vi "Main_18b.vi"() -> ()   [LabVIEW 2023]
uses:
  Cluster_Location.ctl
panel:
  out "MAX Surfaces":i32
  out "number of Blocks":i32
  in  "Example 2":string="2,2,2\n1,2,2\n3,2,2\n2,1,2\n2,3,2\n2,2,1\n2,2,3\n2,2,4\n2,2,6\n1,2,5\n3,2,5\n2,1,5\n2,3,5"
  out "z":i32
  out "x":i32
  out "y":i32
  out "Answer":i32
  in  "Puzzle":string="8,17,5\n6,17,7\n8,9,2\n13,5,16\n5,3,9\n19,4,10\n5,14,5\n3,5,12\n4,6,13\n11,9,3\n11,2,14\n3,14,10\n12,1,11\n16,16,13\n1,9,10\n11,9,19\n15,15,12\n10,4,6\n4,12,17\n17,6,15\n19,14,13\n9,13,2\n18,8,14\n17,7,15\n10,5,17\n14,8,17\n11,19,13\n13,3,14\n8,5,10\n8,16,6\n10,7,20\n7,17,5\n12,18,13\n4,8,13\n3,13,13\n4,3,11\n4,9,15\n17,6,7\n13,5,14\n3,12,7\n13,18,7\n1,9,11\n17,8,15\n12,8,2\n4,9,6\n3,7,12\n8,13,4\n3,8,7\n14,7,3\n16,7,14\n17,5,12\n13,8,2\n17,5,5\n16,5,13\n5,4,13\n6,1,9\n1,11,10\n5,13,5\n10,17,5\n6,3,9\n15,6,7\n11,15,17\n18,6,12\n8,3,11\n14,7,14\n10,6,18\n12,11,4\n3,7,15\n7,3,10\n18,8,13\n16,11,19\n11,3,11\n3,15,14\n16,14,3\n19,10,8\n8,13,18\n15,10,3\n20,7,12\n13,15,16\n18,10,9\n10,2,7\n16,5,12\n6,10,18\n12,19,13\n6,5,6\n14,2,8\n4,16,9\n6,17,9\n15,6,5\n9,4,3\n11,7,2\n19,9,6\n14,12,2\n15,6,18\n18,13,7\n5,6,6\n20,11,14\n19,10,10\n18,10,6\n6,10,5\n16,10,18\n3,9,7\n13,2,7\n14,9,19\n9,14,19\n7,18,6\n8,9,19\n11,1,13\n15,17,10\n2,12,13\n5,17,14\n18,9,11\n15,18,15\n7,3,11\n10,18,6\n17,15,14\n17,7,8\n7,3,14\n7,11,19\n7,9,3\n17,11,6\n16,3,10\n9,18,16\n13,1,10\n15,12,16\n14,12,20\n11,2,8\n18,5,9\n11,16,3\n18,10,7\n4,12,6\n5,11,18\n3,14,14\n16,4,12\n8,3,4\n6,14,3\n17,9,18\n2,11,7\n19,15,12\n13,17,15\n10,7,3\n1,11,8\n18,12,16\n18,12,9\n7,4,4\n12,2,7\n7,14,15\n15,13,3\n3,7,11\n12,17,10\n17,5,14\n5,18,11\n5,4,11\n4,15,15\n8,19,12\n18,12,10\n9,3,11\n3,14,12\n18,7,16\n10,9,19\n16,3,11\n15,11,17\n18,7,12\n9,8,19\n3,15,12\n17,4,12\n5,16,7\n8,4,5\n2,7,11\n5,15,17\n9,20,12\n5,11,4\n4,5,9\n4,15,11\n14,14,5\n11,3,6\n12,3,15\n5,6,10\n5,9,5\n18,15,12\n4,12,5\n19,9,15\n4,6,11\n1,14,9\n5,16,15\n9,3,7\n16,10,4\n17,12,7\n18,8,7\n14,5,9\n6,6,14\n5,14,15\n6,7,3\n18,15,15\n12,7,17\n5,14,16\n6,11,3\n6,10,16\n3,7,8\n10,7,4\n8,8,3\n11,4,5\n16,13,18\n13,6,4\n10,17,16\n3,16,10\n10,19,13\n15,5,16\n9,19,6\n9,13,4\n17,16,7\n12,4,15\n7,4,15\n18,17,10\n14,17,7\n13,15,19\n4,10,15\n13,18,17\n14,19,10\n18,10,15\n14,18,8\n16,4,13\n17,14,9\n14,17,5\n6,7,4\n5,9,16\n5,14,17\n14,19,11\n6,18,7\n14,9,18\n17,7,16\n4,10,16\n11,13,3\n3,10,16\n8,9,18\n13,3,15\n17,8,6\n3,13,9\n5,17,10\n14,15,3\n15,5,15\n16,17,15\n9,20,8\n8,2,13\n20,8,8\n17,14,12\n5,7,18\n5,10,16\n3,8,11\n3,11,16\n15,7,5\n17,12,18\n10,19,11\n11,2,10\n18,11,6\n5,11,17\n15,10,15\n18,15,9\n7,5,15\n17,8,5\n5,5,6\n17,14,16\n15,11,5\n8,10,19\n3,13,14\n7,3,9\n13,2,8\n17,9,6\n17,16,11\n11,10,18\n12,17,18\n5,3,14\n12,9,2\n5,14,6\n14,15,15\n15,4,9\n8,12,17\n10,9,3\n4,17,9\n1,11,12\n3,14,11\n11,19,9\n12,17,8\n5,5,9\n19,9,12\n16,4,14\n18,10,14\n8,19,13\n11,3,8\n6,6,4\n13,6,18\n6,14,4\n18,6,8\n4,13,15\n11,7,1\n11,7,18\n10,3,7\n14,15,7\n6,16,9\n14,7,19\n12,6,17\n16,12,5\n3,10,7\n7,12,5\n16,10,15\n17,8,11\n10,18,14\n3,11,4\n7,10,19\n10,4,3\n12,16,6\n9,8,1\n10,4,15\n14,4,5\n5,8,16\n8,13,3\n19,10,9\n17,17,13\n4,5,11\n14,5,16\n16,11,17\n17,7,6\n1,10,11\n11,8,16\n4,15,6\n10,19,14\n6,4,9\n18,11,8\n10,4,5\n11,13,19\n13,6,16\n5,10,17\n3,11,5\n18,17,9\n18,14,11\n10,1,7\n15,9,3\n8,6,3\n6,3,12\n12,2,8\n14,16,17\n16,8,4\n15,7,4\n19,15,9\n17,16,9\n7,14,19\n3,10,8\n9,20,13\n8,8,1\n5,12,4\n8,17,15\n17,3,10\n16,8,6\n18,10,5\n15,8,5\n6,12,4\n1,16,10\n15,17,6\n20,11,11\n4,4,14\n9,9,3\n6,15,17\n16,9,17\n12,12,19\n19,8,10\n4,14,17\n9,15,17\n10,3,14\n4,6,7\n2,8,12\n13,2,11\n7,11,2\n10,19,7\n15,10,2\n6,13,3\n11,10,20\n6,12,18\n15,18,13\n10,8,2\n13,5,5\n11,2,9\n6,17,14\n6,8,5\n14,14,16\n6,8,16\n3,12,16\n8,17,18\n12,2,11\n3,15,11\n10,11,2\n11,17,12\n9,15,3\n6,16,17\n18,6,6\n16,12,16\n7,18,12\n17,15,4\n9,12,18\n17,6,6\n11,8,19\n12,8,3\n20,9,14\n4,12,16\n20,11,10\n4,15,8\n4,7,9\n16,7,5\n10,9,18\n2,11,12\n4,13,16\n9,2,10\n16,7,18\n17,11,16\n6,15,4\n7,18,7\n6,9,19\n8,15,4\n5,16,14\n2,10,7\n8,12,4\n14,18,13\n12,14,17\n15,11,19\n6,13,16\n14,7,18\n19,11,7\n6,17,16\n10,11,3\n7,20,13\n10,18,7\n8,17,6\n4,7,16\n8,3,15\n2,10,9\n5,3,13\n17,10,15\n9,4,6\n8,19,11\n9,16,4\n14,8,19\n13,12,15\n4,13,17\n14,16,5\n5,6,16\n14,13,17\n18,7,13\n12,3,6\n6,4,14\n10,4,9\n3,10,6\n8,19,9\n11,7,19\n19,12,14\n18,9,10\n16,10,17\n16,6,16\n17,15,15\n7,18,11\n1,10,12\n12,4,13\n8,5,5\n20,10,12\n9,18,8\n18,13,9\n8,17,4\n18,7,6\n7,13,4\n15,17,14\n11,17,17\n4,11,16\n7,5,17\n8,15,17\n14,18,6\n15,12,3\n2,7,13\n11,5,5\n19,14,11\n15,18,9\n11,18,5\n7,6,6\n10,11,19\n8,14,3\n6,13,17\n12,5,15\n16,9,3\n3,5,6\n10,4,16\n14,13,19\n3,6,12\n9,15,14\n17,13,7\n7,19,11\n8,14,16\n3,17,12\n9,11,18\n18,14,7\n17,17,9\n8,13,2\n4,16,15\n11,15,4\n8,4,9\n13,6,17\n4,7,12\n13,3,10\n6,5,9\n5,6,5\n15,14,5\n11,4,6\n4,17,13\n3,11,11\n16,13,5\n12,9,1\n13,9,18\n8,17,9\n5,11,15\n16,14,5\n13,11,19\n10,16,17\n9,12,3\n3,12,10\n6,9,4\n5,13,15\n11,6,18\n16,4,9\n7,12,3\n18,12,6\n10,16,18\n14,6,18\n4,5,7\n6,8,18\n15,10,18\n8,3,13\n10,5,18\n3,6,15\n14,6,16\n14,6,17\n12,10,3\n2,14,12\n18,5,10\n15,9,17\n8,6,18\n3,16,14\n10,13,4\n10,15,19\n4,8,17\n13,6,5\n3,6,10\n12,20,10\n11,6,4\n18,4,11\n17,9,11\n15,4,13\n9,17,5\n6,3,11\n11,19,6\n17,6,14\n7,7,18\n8,10,2\n9,3,15\n4,16,13\n11,5,15\n3,6,13\n8,15,18\n14,3,14\n6,5,14\n5,12,18\n8,3,12\n15,4,16\n6,6,15\n16,16,9\n15,3,14\n8,14,18\n10,17,6\n5,9,6\n15,8,16\n18,6,5\n15,13,4\n15,16,5\n10,7,5\n9,7,18\n16,3,13\n4,8,4\n11,11,19\n17,13,12\n17,11,15\n4,13,14\n10,2,6\n4,10,4\n10,3,6\n9,16,17\n8,1,9\n14,20,9\n3,7,14\n8,18,16\n3,11,14\n16,14,15\n3,10,9\n17,12,12\n3,14,5\n10,16,3\n5,15,13\n15,16,7\n12,16,19\n2,12,11\n2,13,10\n13,18,14\n16,15,18\n2,10,15\n2,8,8\n6,7,6\n13,5,17\n6,4,15\n9,17,6\n5,16,13\n11,5,18\n7,17,10\n17,6,5\n14,4,12\n8,12,20\n2,15,10\n18,6,13\n12,19,16\n19,7,5\n19,9,14\n10,13,18\n6,11,19\n10,14,3\n19,7,11\n7,18,16\n14,9,2\n12,4,5\n15,14,6\n5,9,17\n11,14,2\n15,13,18\n16,16,8\n2,5,9\n2,8,10\n16,5,6\n6,18,10\n12,18,15\n4,14,12\n15,8,17\n18,9,9\n11,10,1\n12,3,3\n9,19,9\n8,5,13\n20,14,12\n16,5,15\n1,12,10\n19,15,11\n13,17,10\n12,2,5\n3,5,10\n7,6,5\n5,7,4\n9,6,18\n16,17,12\n7,8,19\n17,11,12\n10,18,15\n13,16,15\n2,12,14\n8,12,2\n14,18,7\n17,5,9\n3,13,5\n10,14,19\n3,8,13\n16,15,3\n11,6,20\n3,14,8\n14,8,18\n7,17,12\n4,13,5\n17,7,5\n8,7,17\n14,4,6\n17,12,4\n13,3,6\n10,12,3\n9,21,11\n17,11,13\n2,16,13\n7,5,3\n14,16,16\n17,15,6\n14,3,13\n11,3,13\n16,16,15\n13,2,13\n17,14,15\n12,2,15\n17,14,11\n10,14,4\n6,8,4\n16,7,15\n11,4,17\n17,17,11\n12,4,17\n6,9,15\n12,9,20\n16,11,5\n18,5,7\n8,11,18\n15,12,6\n12,13,3\n7,15,3\n5,11,3\n11,16,8\n16,17,14\n4,8,7\n14,5,7\n4,13,18\n15,17,7\n16,15,17\n14,20,11\n10,6,14\n12,19,10\n13,3,16\n13,18,8\n13,19,10\n10,10,3\n9,2,8\n6,16,16\n6,16,7\n13,17,5\n3,8,12\n12,13,17\n13,19,12\n19,13,8\n6,10,17\n16,16,7\n7,14,6\n5,15,6\n13,1,12\n7,3,13\n11,17,6\n13,15,3\n10,2,12\n14,2,13\n19,11,6\n8,8,17\n4,6,6\n4,16,10\n4,5,12\n14,19,14\n17,15,16\n11,15,18\n10,15,3\n8,2,10\n15,9,8\n17,13,16\n2,13,14\n15,7,6\n10,12,20\n4,17,14\n12,6,16\n18,7,7\n5,9,4\n16,15,7\n18,16,10\n10,2,10\n13,17,17\n15,6,12\n10,7,2\n11,0,12\n13,2,6\n17,9,5\n10,16,5\n19,10,13\n7,11,16\n5,17,13\n8,18,13\n15,7,19\n3,12,8\n7,18,15\n12,17,3\n16,5,16\n9,16,16\n14,5,15\n8,2,9\n7,16,7\n12,5,16\n19,8,15\n17,10,16\n9,5,6\n12,7,4\n3,4,9\n11,14,19\n12,12,1\n15,12,4\n16,12,17\n18,10,12\n19,12,6\n15,8,15\n12,19,14\n3,8,6\n14,2,12\n11,5,4\n10,5,3\n9,11,3\n7,12,19\n3,5,7\n20,7,11\n15,3,12\n13,4,9\n13,14,2\n17,13,14\n16,4,11\n10,3,17\n15,16,8\n18,16,8\n4,14,14\n11,19,8\n5,11,6\n9,3,16\n10,17,7\n13,9,19\n5,13,8\n12,4,4\n8,13,1\n7,2,11\n6,6,5\n9,5,3\n12,14,3\n14,3,11\n10,6,4\n8,16,18\n10,18,17\n9,7,2\n6,5,8\n10,2,13\n17,8,16\n6,3,10\n7,13,18\n8,18,14\n4,9,17\n12,7,19\n3,12,11\n16,16,14\n4,14,13\n9,5,5\n4,6,16\n7,16,16\n12,15,17\n19,16,11\n8,9,16\n1,13,13\n16,15,5\n2,11,8\n6,2,12\n9,5,15\n12,2,13\n8,13,19\n15,5,7\n7,19,9\n7,1,8\n17,8,4\n5,5,4\n5,4,12\n11,12,3\n8,15,3\n16,16,12\n16,13,17\n5,6,8\n10,10,2\n4,16,14\n10,8,20\n3,9,16\n5,12,5\n7,16,6\n18,6,14\n6,5,17\n2,7,8\n16,17,11\n12,3,12\n11,4,16\n17,11,5\n13,4,11\n15,6,8\n6,10,6\n11,1,10\n10,19,12\n3,14,13\n12,18,9\n7,15,5\n10,3,9\n10,8,18\n16,14,4\n20,9,9\n10,15,2\n10,5,16\n10,17,4\n14,11,2\n15,9,4\n15,3,9\n15,6,17\n2,9,11\n7,13,17\n6,17,15\n16,12,4\n16,5,7\n11,5,17\n5,12,7\n10,3,13\n6,10,4\n17,10,4\n6,4,10\n14,18,14\n12,18,10\n13,18,6\n15,6,13\n15,16,12\n16,6,12\n17,10,7\n17,10,5\n1,9,12\n3,9,5\n17,15,7\n13,13,4\n4,5,13\n15,12,2\n13,4,4\n15,13,17\n19,12,10\n15,18,7\n12,17,17\n16,7,4\n19,7,12\n3,12,5\n11,19,12\n10,20,9\n13,15,18\n18,6,11\n9,1,10\n12,8,20\n18,13,10\n2,12,15\n3,6,11\n14,8,16\n7,10,5\n4,13,6\n10,14,1\n7,12,18\n10,18,11\n2,11,13\n6,6,6\n17,4,8\n13,4,16\n5,14,9\n18,12,5\n4,12,12\n18,15,11\n12,17,4\n17,7,11\n12,17,15\n13,10,1\n2,15,9\n4,10,5\n6,14,6\n15,7,7\n6,16,12\n15,9,2\n12,2,12\n9,4,5\n3,14,7\n9,15,5\n4,7,8\n8,16,17\n19,6,9\n19,8,7\n13,3,9\n14,13,15\n7,17,14\n8,4,12\n13,18,9\n6,5,15\n17,5,6\n13,13,3\n13,17,13\n13,6,2\n11,3,9\n3,8,14\n7,4,8\n4,14,6\n8,5,18\n13,7,18\n13,7,3\n14,11,17\n7,5,16\n13,3,12\n19,12,15\n14,3,5\n17,11,18\n9,3,10\n15,7,3\n2,9,12\n6,18,9\n3,6,9\n13,19,7\n18,11,7\n3,15,8\n2,12,12\n16,15,11\n4,4,11\n6,7,11\n1,10,13\n15,3,11\n14,18,10\n6,9,18\n18,9,15\n12,19,11\n7,6,7\n3,12,18\n3,11,9\n14,17,6\n16,16,11\n18,14,14\n8,20,11\n18,6,7\n15,6,16\n5,9,3\n14,2,14\n10,7,18\n7,4,17\n20,6,9\n15,5,10\n15,4,12\n20,10,15\n6,12,2\n10,4,4\n5,15,15\n5,16,10\n6,11,2\n10,13,2\n7,15,4\n15,16,4\n16,5,8\n4,6,15\n8,5,14\n4,17,12\n6,14,5\n11,17,7\n15,14,15\n17,12,5\n6,18,13\n16,17,9\n7,7,16\n4,6,9\n7,10,3\n16,14,12\n19,12,12\n15,17,9\n13,2,12\n6,9,3\n12,3,9\n15,14,3\n14,14,19\n14,8,3\n9,8,18\n4,13,7\n10,4,8\n8,1,7\n5,5,13\n14,3,16\n6,20,9\n6,15,18\n5,14,18\n19,9,8\n5,2,12\n16,8,15\n10,3,8\n13,15,4\n8,16,3\n13,13,2\n14,18,12\n16,5,14\n11,14,18\n5,7,5\n8,9,20\n9,8,3\n16,16,6\n13,20,9\n11,18,14\n15,13,5\n11,14,17\n12,17,6\n10,17,15\n6,8,15\n2,7,12\n12,20,13\n9,14,17\n12,16,5\n10,19,6\n7,7,4\n1,11,11\n19,6,10\n15,14,4\n19,13,12\n4,7,6\n9,2,12\n9,19,15\n18,14,16\n11,10,2\n13,16,4\n17,12,15\n2,10,10\n2,13,13\n5,10,3\n10,16,7\n11,19,10\n17,14,8\n12,12,20\n7,5,8\n11,8,20\n5,15,8\n3,9,8\n13,5,13\n17,15,10\n14,11,19\n15,5,4\n15,3,8\n15,4,6\n4,15,14\n17,11,17\n12,6,15\n3,16,7\n4,11,5\n13,10,3\n7,14,3\n6,17,12\n14,16,4\n4,16,12\n4,14,5\n14,19,9\n19,13,9\n10,10,19\n11,11,1\n18,16,12\n17,17,8\n10,12,2\n7,18,8\n1,8,12\n19,8,6\n4,6,8\n13,14,17\n20,10,8\n19,7,7\n12,3,14\n2,9,8\n5,17,11\n11,8,2\n7,18,9\n8,7,3\n9,15,18\n10,6,16\n7,16,3\n15,8,18\n11,14,3\n17,13,6\n11,8,18\n14,5,5\n17,16,14\n17,13,4\n9,7,17\n13,5,6\n14,3,12\n3,13,16\n11,3,7\n16,10,16\n11,16,4\n7,3,15\n5,16,11\n20,9,10\n18,8,9\n19,8,8\n20,9,13\n11,16,16\n15,11,2\n1,13,12\n14,13,4\n12,18,11\n14,16,3\n11,5,11\n17,7,13\n15,11,18\n7,17,9\n5,5,14\n11,9,2\n4,7,14\n7,17,15\n5,12,17\n3,8,15\n18,10,16\n15,4,11\n12,5,6\n19,11,11\n11,18,17\n18,13,16\n7,4,7\n7,5,6\n13,10,19\n13,18,10\n16,15,16\n5,7,15\n12,12,2\n2,14,8\n20,9,11\n4,7,11\n5,11,12\n16,16,10\n3,17,9\n2,9,9\n17,18,9\n3,12,15\n5,3,11\n15,4,15\n20,10,14\n19,13,11\n5,13,18\n17,9,4\n13,12,17\n3,15,13\n14,10,6\n16,16,5\n5,8,17\n15,3,6\n18,15,10\n15,6,6\n18,11,14\n17,12,13\n4,6,14\n5,14,3\n15,5,6\n11,15,3\n12,2,9\n14,3,15\n17,12,16\n15,17,13\n13,12,1\n14,3,10\n18,9,14\n12,17,11\n16,11,15\n18,8,6\n3,12,6\n3,9,6\n7,16,8\n16,12,15\n18,8,10\n4,5,10\n12,19,7\n14,2,9\n8,7,6\n12,3,11\n4,7,7\n9,18,14\n4,6,5\n11,17,16\n8,19,10\n12,8,19\n3,17,13\n15,12,18\n4,4,13\n10,19,8\n16,8,17\n9,7,16\n19,14,9\n9,8,2\n16,8,13\n7,5,14\n7,6,4\n18,11,10\n6,4,5\n18,7,14\n18,11,13\n9,6,3\n8,16,15\n7,8,3\n12,9,3\n9,19,7\n8,6,16\n10,4,17\n17,4,14\n11,13,18\n6,8,17\n3,7,17\n16,4,8\n2,10,8\n5,18,8\n9,3,6\n18,9,5\n9,15,19\n3,16,9\n7,6,17\n7,16,17\n12,11,19\n12,10,2\n4,7,10\n6,19,13\n19,11,10\n9,10,1\n12,14,4\n4,9,4\n18,16,9\n5,3,8\n9,18,4\n3,13,6\n16,15,14\n13,8,19\n12,16,14\n8,10,15\n11,21,12\n5,15,5\n8,9,15\n18,11,5\n16,17,8\n10,17,17\n11,8,3\n7,19,12\n14,16,8\n17,15,12\n11,11,4\n7,6,19\n3,16,12\n17,5,10\n11,3,16\n8,15,14\n8,15,5\n2,9,13\n5,11,5\n4,4,8\n12,5,17\n7,5,7\n6,19,11\n4,7,4\n17,9,7\n15,7,16\n9,14,3\n14,4,15\n16,7,17\n3,12,9\n17,9,16\n8,18,10\n11,16,5\n10,18,8\n14,5,6\n12,15,16\n10,6,19\n14,7,17\n2,14,11\n8,5,8\n16,9,4\n8,3,7\n8,3,14\n19,9,13\n6,8,3\n17,14,17\n13,3,13\n4,13,4\n3,10,14\n17,16,12\n17,5,11\n12,3,10\n15,8,3\n17,9,14\n14,7,4\n5,9,18\n10,2,9\n13,4,7\n7,15,17\n11,13,20\n8,18,7\n12,13,20\n17,16,13\n10,6,2\n3,6,5\n7,2,13\n12,4,16\n14,15,18\n12,9,17\n8,12,18\n7,10,2\n17,3,8\n9,3,9\n14,9,3\n10,3,10\n14,6,5\n16,14,10\n6,3,13\n9,19,12\n19,9,11\n9,9,19\n17,15,13\n19,6,13\n10,3,12\n15,4,14\n10,5,5\n6,12,16\n10,11,18\n4,9,5\n19,15,8\n4,15,7\n14,16,14\n12,1,9\n9,14,2\n12,15,3\n14,10,17\n15,15,17\n14,4,10\n3,13,12\n17,17,10\n9,17,4\n3,9,11\n11,15,13\n20,11,8\n18,13,13\n3,11,8\n14,3,7\n18,11,12\n19,14,8\n18,13,6\n10,16,16\n9,1,12\n5,8,13\n11,2,13\n2,15,8\n11,3,14\n8,17,14\n8,6,6\n5,13,4\n5,15,4\n4,3,7\n14,17,14\n12,15,2\n13,5,4\n14,15,4\n15,14,16\n19,12,9\n19,8,11\n7,11,3\n3,5,13\n6,13,19\n15,13,6\n11,6,17\n18,8,8\n11,18,10\n10,12,18\n2,10,12\n18,9,17\n18,7,8\n7,16,11\n9,20,11\n17,13,17\n9,14,1\n4,4,12\n6,19,10\n2,9,14\n18,11,11\n18,5,13\n3,7,13\n13,12,2\n13,17,6\n2,7,9\n18,8,11\n4,16,11\n7,7,5\n14,17,16\n12,3,5\n11,17,18\n15,16,16\n9,13,19\n17,14,14\n6,17,6\n13,4,5\n5,8,18\n9,11,20\n17,10,8\n8,16,2\n17,7,7\n14,14,17\n15,7,14\n14,10,19\n6,11,5\n15,8,4\n9,3,14\n5,14,4\n4,11,4\n15,16,11\n7,16,14\n8,18,12\n17,12,6\n6,9,17\n13,15,17\n4,4,9\n8,7,18\n12,19,9\n16,14,17\n2,7,7\n7,14,18\n18,12,15\n5,17,9\n6,2,9\n12,19,15\n5,7,17\n16,15,15\n13,3,11\n8,2,11\n11,4,8\n10,12,21\n9,15,16\n3,7,9\n10,2,11\n4,8,6\n17,10,6\n11,3,17\n4,11,18\n11,4,3\n4,11,8\n18,5,8\n12,13,2\n14,4,4\n13,11,18\n8,14,2\n6,7,16\n20,11,13\n12,3,7\n4,11,10\n6,3,6\n12,18,7\n8,5,11\n15,2,11\n17,5,7\n18,14,9\n9,4,11\n13,11,3\n10,19,10\n18,14,8\n16,11,4\n10,4,11\n10,8,19\n13,18,5\n10,9,1\n13,20,10\n6,8,6\n10,14,2\n18,8,5\n9,14,18\n3,8,8\n16,9,16\n17,8,14\n9,6,16\n7,9,20\n3,13,11\n17,8,13\n18,10,4\n16,6,9\n12,19,8\n6,15,6\n8,8,4\n7,14,4\n13,17,14\n19,6,6\n4,17,11\n8,17,16\n12,9,19\n2,11,11\n19,8,13\n6,5,5\n9,17,16\n14,4,9\n17,8,9\n4,13,9\n2,8,13\n17,4,10\n13,8,16\n2,13,11\n5,5,11\n15,9,19\n11,15,19\n7,17,18\n7,3,7\n13,16,16\n8,17,12\n15,2,14\n9,9,2\n7,4,13\n7,18,14\n5,16,5\n17,16,8\n11,1,7\n4,11,13\n18,11,9\n4,15,10\n2,7,10\n12,10,18\n7,10,16\n14,3,6\n20,10,11\n4,8,11\n6,15,5\n3,12,13\n5,4,10\n2,9,7\n16,5,9\n13,5,3\n15,7,17\n6,16,11\n9,18,15\n10,20,10\n13,8,18\n19,10,12\n5,6,17\n17,10,3\n15,11,3\n18,12,11\n13,4,6\n13,14,16\n2,12,10\n6,14,18\n15,16,6\n10,18,10\n4,14,16\n3,13,7\n13,8,20\n10,18,5\n12,2,10\n18,5,11\n15,2,6\n13,7,2\n10,3,15\n10,15,16\n4,6,12\n20,12,7\n8,3,10\n16,4,10\n20,13,8\n17,3,12\n13,11,4\n8,3,8\n7,3,6\n5,17,8\n18,13,11\n14,11,16\n5,11,16\n11,16,6\n16,9,5\n4,3,9\n14,4,16\n5,10,4\n7,2,10\n14,4,8\n14,17,9\n4,5,15\n15,15,5\n6,17,8\n5,3,12\n3,14,9\n8,12,19\n5,7,11\n18,7,15\n9,5,2\n13,10,17\n7,9,18\n19,7,13\n3,7,6\n13,9,2\n4,10,13\n10,14,17\n3,12,12\n12,7,18\n16,6,7\n15,8,19\n9,15,4\n12,7,2\n14,13,18\n6,4,11\n3,7,5\n18,9,13\n17,3,11\n5,4,15\n9,16,3\n13,10,2\n16,19,10\n19,14,10\n13,2,14\n9,3,13\n12,18,12\n15,18,12\n10,20,14\n6,7,18\n13,8,3\n6,11,20\n8,4,10\n11,3,10\n5,6,13\n8,2,12\n2,9,10\n3,12,14\n2,12,7\n18,6,15\n15,13,19\n16,15,9\n17,5,8\n7,6,18\n7,2,7\n19,7,9\n17,6,12\n6,19,14\n5,16,17\n6,10,3\n7,12,4\n17,15,11\n12,8,18\n2,14,13\n5,8,6\n15,4,10\n7,7,17\n19,9,9\n16,14,8\n16,7,13\n11,10,3\n14,11,1\n16,15,12\n5,15,7\n7,3,8\n12,3,13\n11,3,15\n9,3,5\n13,2,10\n19,11,9\n11,12,20\n8,8,2\n7,9,19\n19,13,14\n18,9,6\n18,15,14\n5,6,14\n20,5,9\n8,4,15\n8,16,5\n2,6,11\n8,4,4\n6,19,9\n7,18,10\n14,8,4\n9,18,7\n9,6,19\n9,5,16\n18,15,7\n16,16,16\n8,12,3\n5,16,9\n5,6,15\n15,6,4\n8,2,14\n9,13,1\n2,14,7\n11,16,2\n9,18,6\n18,9,16\n17,15,8\n6,13,14\n14,4,11\n9,12,2\n11,16,18\n9,4,9\n15,15,6\n9,8,17\n5,12,6\n16,8,3\n15,14,2\n6,18,14\n18,16,14\n14,7,6\n16,3,9\n15,6,14\n10,15,18\n7,5,4\n12,3,16\n9,6,14\n6,18,15\n18,15,8\n6,15,7\n16,3,8\n2,13,8\n9,16,5\n8,7,16\n18,11,17\n17,9,17\n17,8,17\n17,12,17\n16,6,6\n8,11,3\n5,13,14\n8,2,8\n15,17,11\n5,6,9\n2,11,9\n11,2,11\n5,18,12\n18,16,11\n6,9,8\n12,5,4\n1,8,8\n6,14,17\n12,8,1\n13,3,7\n2,10,13\n7,13,3\n17,14,13\n15,18,14\n7,17,7\n13,15,2\n9,2,13\n6,2,10\n6,14,14\n15,14,12\n8,2,15\n13,11,2\n4,15,13\n18,12,14\n16,17,7\n20,10,9\n16,15,6\n12,11,3\n6,18,12\n11,4,4\n18,11,16\n17,12,9\n3,8,5\n7,4,6\n13,4,13\n18,9,7\n15,5,12\n2,13,12\n14,3,9\n3,6,8\n16,8,11\n11,12,18\n19,12,13\n16,15,4\n13,16,6\n4,9,7\n12,9,5\n15,7,18\n15,10,5\n19,5,10\n10,2,8\n10,4,14\n17,4,11\n19,14,12\n3,11,13\n8,18,9\n1,10,9\n6,4,7\n12,7,3\n2,15,11\n13,19,11\n14,17,10\n2,5,12\n11,20,10\n4,7,17\n10,17,8\n7,11,18\n4,10,17\n13,12,20\n7,8,4\n19,13,13\n4,5,8\n13,6,19\n5,12,3\n5,16,6\n13,4,12\n9,11,2\n15,15,2\n5,16,8\n8,3,16\n13,4,15\n14,12,4\n13,16,5\n14,15,5\n4,7,5\n6,4,13\n11,18,8\n12,17,5\n7,2,9\n14,2,11\n10,10,20\n9,10,20\n17,15,9\n12,14,18\n8,11,19\n19,7,14\n10,13,19\n12,10,19\n6,20,11\n5,8,15\n7,2,8\n9,12,20\n8,13,16\n2,14,6\n3,10,5\n16,7,6\n7,2,12\n6,16,6\n13,7,4\n14,9,17\n9,19,8\n3,5,11\n17,4,9\n16,15,8\n10,5,6\n9,1,9\n6,4,16\n19,12,11\n6,9,5\n11,17,10\n10,19,15\n9,15,2\n3,17,8\n20,13,11\n15,4,7\n7,17,16\n8,16,7\n18,9,12\n3,10,12\n4,14,10\n4,5,14\n4,6,10\n15,17,15\n11,11,3\n12,2,14\n9,7,3\n9,3,8\n13,20,13\n4,12,4\n8,4,7\n16,6,10\n19,10,7\n6,3,15\n5,7,16\n9,1,15\n8,1,11\n4,8,15\n8,11,20\n8,16,4\n13,1,9\n11,6,3\n6,11,4\n15,16,14\n5,4,14\n10,20,11\n14,2,10\n19,11,12\n18,12,13\n7,10,18\n3,14,15\n4,12,9\n5,8,4\n8,20,9\n13,5,15\n14,19,13\n18,9,8\n10,12,19\n4,13,11\n4,18,14\n16,5,10\n12,4,6\n16,8,8\n6,5,4\n11,4,18\n7,4,9\n9,5,17\n17,9,15\n16,12,12\n16,18,9\n5,5,10\n3,5,8\n4,10,14\n6,15,16\n8,1,10\n17,14,10\n15,10,4\n11,9,20\n5,7,3\n13,7,16\n12,10,20\n18,10,10\n4,10,10\n7,4,3\n15,9,18\n11,12,4\n8,10,17\n4,19,10\n8,19,8\n16,9,2\n11,2,7\n11,7,17\n10,8,3\n9,11,19\n7,13,2\n11,17,4\n10,12,1\n5,5,8\n13,13,19\n16,18,15\n6,16,8\n15,17,16\n15,10,17\n13,15,15\n11,3,12\n13,12,18\n7,16,5\n12,11,1\n19,7,10\n7,3,12\n19,12,7\n18,16,7\n13,14,3\n15,13,2\n8,6,4\n8,6,15\n5,14,11\n3,9,14\n8,5,4\n14,12,16\n19,8,12\n10,7,19\n9,16,18\n11,18,13\n15,16,17\n3,9,13\n10,13,1\n16,13,4\n8,11,1\n14,5,3\n12,6,18\n18,8,15\n11,18,11\n4,14,8\n5,12,15\n2,8,9\n3,10,13\n6,12,17\n3,6,14\n8,7,4\n16,8,18\n4,5,5\n4,8,9\n16,19,11\n13,3,8\n6,6,17\n4,12,13\n8,17,17\n10,13,3\n16,16,4\n12,6,5\n7,19,13\n18,14,12\n14,6,3\n17,7,12\n17,16,10\n2,12,9\n1,12,12\n11,13,17\n15,17,8\n11,3,5\n14,4,14\n9,4,13\n12,16,17\n5,17,7\n18,4,10\n12,18,5\n3,15,10\n9,10,19\n6,10,2\n10,6,1\n6,12,3\n13,4,17\n15,15,16\n5,15,12\n15,15,14\n11,2,5\n12,5,3\n14,18,11\n15,16,15\n11,19,7\n3,11,7\n5,9,14\n9,1,13\n15,18,11\n14,12,3\n11,20,9\n2,13,15\n4,18,12\n10,4,7\n19,13,10\n11,20,12\n9,8,16\n12,18,14\n9,18,13\n12,16,15\n17,5,13\n11,2,6\n9,4,17\n7,17,13\n11,6,15\n18,13,14\n9,17,15\n12,11,2\n16,17,13\n6,16,4\n14,14,3\n19,10,11\n16,6,5\n10,18,4\n6,13,2\n18,9,4\n10,9,2\n13,16,17\n13,18,15\n7,17,11\n6,13,4\n1,12,13\n11,1,12\n18,14,10\n7,19,14\n10,3,16\n10,21,12\n15,19,10\n9,13,3\n13,7,17\n8,11,2\n6,5,7\n6,13,5\n13,17,8\n15,4,8\n19,10,6\n2,11,6\n10,19,9\n5,4,7\n10,17,13\n6,13,18\n8,7,19\n2,12,8\n9,2,6\n12,6,19\n13,12,3\n7,4,11\n3,13,17\n10,2,5\n20,7,8\n14,4,7\n13,17,4\n14,18,15\n15,6,15\n8,17,8\n3,9,9\n17,18,7\n5,7,7\n3,11,12\n17,6,13\n4,11,7\n17,8,18\n5,14,14\n5,6,4\n6,18,11\n17,3,13\n3,13,8\n5,7,6\n1,13,10\n5,13,16\n19,7,8\n4,11,17\n6,17,13\n15,17,5\n18,13,8\n18,8,16\n1,8,13\n4,9,12\n12,15,18\n7,13,5\n9,18,17\n11,6,16\n13,4,14\n9,4,4\n10,17,14\n13,14,18\n12,15,19\n6,12,6\n7,19,10\n1,12,9\n20,10,13\n14,14,15\n12,15,4\n4,12,15\n5,10,18\n10,8,17\n6,6,3\n3,10,10\n5,18,7\n7,12,17\n8,15,2\n12,14,20\n11,16,17\n4,14,15\n13,20,8\n4,11,14\n7,16,15\n9,19,14\n9,6,20\n3,16,8\n10,1,8\n11,13,1\n14,1,11\n16,18,10\n1,11,9\n14,20,10\n9,19,13\n10,20,12\n3,14,16\n19,6,11\n18,11,15\n19,13,7\n8,18,6\n17,6,16\n16,13,15\n14,15,2\n13,1,8\n6,4,8\n17,6,10\n1,8,10\n15,16,13\n8,19,6\n2,8,11\n7,10,1\n4,16,6\n19,10,15\n19,16,9\n9,10,18\n16,17,6\n16,10,19\n12,1,10\n15,5,5\n2,6,8\n19,8,14\n4,18,11\n10,11,1\n10,21,10\n6,6,16\n5,5,7\n9,5,18\n8,10,3\n12,18,16\n9,2,7\n9,18,5\n5,4,6\n10,11,20\n9,19,11\n12,19,12\n3,11,10\n15,3,13\n7,17,6\n20,11,9\n11,8,17\n11,11,2\n7,4,10\n18,10,8\n13,13,18\n6,8,19\n18,14,15\n6,19,12\n15,12,5\n18,7,9\n8,12,1\n18,6,10\n3,12,4\n10,13,20\n17,15,5\n3,7,7\n7,14,2\n8,4,16\n11,10,21\n11,12,2\n14,19,12\n2,12,6\n16,10,8\n8,17,7\n6,7,5\n11,12,1\n7,13,16\n3,5,14\n12,20,8\n2,10,14\n4,12,7\n8,16,16\n7,4,16\n8,19,16\n9,1,11\n2,10,11\n10,12,17\n19,11,13\n17,14,6\n11,17,15\n3,15,9\n13,19,8\n6,17,10\n12,3,8\n4,4,10\n16,18,6\n6,16,5\n14,4,13\n7,3,17\n16,14,7\n2,16,12\n5,12,16\n6,17,11\n7,10,15\n15,11,4\n10,16,4\n19,11,14\n4,16,8\n6,9,2\n6,16,15\n18,14,6\n7,1,10\n6,5,13\n17,13,15\n20,13,14\n8,9,3\n16,14,11\n17,13,8\n4,17,10\n2,14,9\n8,3,9\n6,15,15\n19,6,8\n4,4,7\n16,3,14\n9,14,16\n4,10,7\n13,3,17\n16,9,18\n9,2,14\n5,17,5\n14,6,2\n15,2,13\n14,17,15\n7,16,12\n10,4,10\n14,19,8\n9,17,7\n6,9,6\n9,12,19\n12,4,18\n15,11,6\n14,5,17\n17,13,10\n9,19,10\n13,2,9\n12,13,19\n15,2,12\n8,14,4\n5,17,12\n19,9,10\n12,6,3\n15,3,5\n9,6,5\n4,12,8\n12,13,18\n8,5,16\n8,4,14\n13,11,20\n14,13,2\n7,12,7\n9,1,7\n15,16,9\n9,9,20\n5,15,14\n12,10,1\n14,17,8\n8,11,17\n10,18,13\n9,4,7\n14,18,9\n12,19,5\n12,1,8\n9,13,18\n5,7,12\n18,6,16\n3,8,9\n18,15,17\n1,10,14\n12,16,4\n14,7,16\n18,10,11\n7,1,13\n14,7,2\n18,13,15\n16,13,16\n11,5,3\n9,5,4\n14,12,18\n12,13,1\n18,15,13\n2,6,10\n4,17,6\n12,1,12\n4,16,7\n12,16,16\n8,18,15\n14,10,18\n9,9,0\n10,1,13\n9,6,4\n12,6,9\n7,7,3\n9,17,14\n17,14,7\n5,18,9\n12,0,11\n16,11,18\n7,14,16\n14,10,3\n13,12,4\n1,11,6\n13,18,11\n3,6,7\n3,15,7\n3,16,13\n19,12,8\n11,15,6\n12,4,8\n8,7,2\n8,10,18\n3,4,13\n7,6,14\n6,12,5\n20,8,12\n3,9,15\n13,14,4\n16,5,5\n5,4,8\n18,15,6\n7,15,18\n7,13,19\n11,8,4\n12,12,17\n14,5,8\n6,7,2\n14,9,20\n16,10,3\n19,11,8\n13,16,18\n15,4,17\n20,12,9\n11,18,16\n5,10,19\n1,9,13\n10,6,17\n3,9,12\n12,17,7\n16,11,6\n5,17,15\n18,13,12\n3,15,15\n10,3,11\n16,5,4\n20,14,11\n5,10,14\n13,17,16\n12,1,13\n10,4,13\n5,5,16\n11,8,1\n16,4,15\n16,17,16\n6,19,8\n11,6,2\n4,18,10\n6,6,7\n14,11,18\n17,10,18\n11,4,13\n14,12,17\n5,16,12\n2,9,6\n12,4,14\n1,14,11\n13,17,3\n5,18,10\n13,15,6\n11,1,9\n11,20,11\n17,10,14\n14,11,3\n14,9,4\n4,3,8\n14,12,5\n12,12,4\n2,6,9\n8,14,19\n4,7,13\n14,12,19\n4,14,7\n18,6,9\n11,12,17\n13,6,3\n12,7,16\n11,2,15\n18,7,5\n5,9,19\n1,8,9\n12,14,16\n5,15,16\n16,18,13\n11,18,9\n15,9,15\n7,5,13\n17,6,8\n17,7,10\n11,18,15\n10,7,1\n2,8,6\n11,13,2\n5,6,11\n7,16,10\n6,5,10\n7,8,2\n8,6,19\n3,13,10\n18,11,4\n17,3,15\n17,11,8\n9,16,6\n15,3,15\n8,5,17\n7,15,8\n15,13,16\n17,4,13\n15,9,16\n16,12,11\n17,12,11\n6,15,13\n2,8,15\n17,7,14\n8,4,6\n17,11,3\n11,20,8\n11,17,14\n8,8,19\n1,12,14\n14,17,11\n7,16,4\n12,14,19\n11,15,20\n8,5,9\n12,11,17\n16,14,6\n11,5,16\n17,9,3\n16,11,16\n3,7,10\n15,3,7\n13,12,5\n7,14,17\n20,12,12\n11,15,2\n3,11,15\n6,12,7\n7,14,5\n17,13,18\n8,5,6\n7,17,4\n4,9,16\n15,18,6\n14,17,17\n10,14,18\n9,4,10\n16,6,11\n11,18,7\n17,12,14\n13,19,6\n14,14,4\n10,20,13\n6,5,11\n7,12,2\n8,15,16\n3,10,11\n4,11,15\n4,9,14\n4,9,10\n10,5,19\n9,2,11\n15,10,19\n10,18,9\n9,9,18\n16,14,16\n4,13,3\n19,11,15\n19,13,16\n16,6,14\n7,2,14\n8,19,7\n16,4,7\n12,11,20\n16,12,18\n10,8,4\n10,5,15\n20,8,13\n4,18,7\n16,6,15\n14,11,4\n10,2,16\n8,8,20\n14,9,16\n7,6,3\n4,8,14\n10,20,8\n7,13,8\n7,17,17\n14,17,12\n2,8,7\n14,2,6\n15,14,17\n4,8,10\n18,5,12\n5,5,15\n11,7,4\n6,18,8\n17,8,3\n7,6,2\n5,14,7\n9,1,14\n10,11,5\n13,18,13\n1,7,12\n8,4,17\n8,18,11\n17,6,11\n12,13,4\n16,4,6\n3,4,11\n5,14,12\n16,18,7\n11,17,13\n9,7,4\n17,13,3\n13,15,5\n8,17,13\n14,8,20\n2,8,14\n15,3,16\n12,19,6\n7,7,19\n6,7,19\n11,10,19\n5,19,9\n7,5,5\n7,9,17\n7,8,17\n16,6,8\n14,16,18\n16,10,7\n4,15,12\n13,20,11\n10,15,4\n14,17,13\n2,15,14\n10,15,17\n7,9,1\n10,17,11\n16,6,13\n17,16,15\n13,17,11\n17,14,5\n7,11,4\n13,5,7\n7,6,16\n14,9,1\n16,15,13\n15,5,14\n3,11,6"
  in  "Example":string="2,2,2\n1,2,2\n3,2,2\n2,1,2\n2,3,2\n2,2,1\n2,2,3\n2,2,4\n2,2,6\n1,2,5\n3,2,5\n2,1,5\n2,3,5"
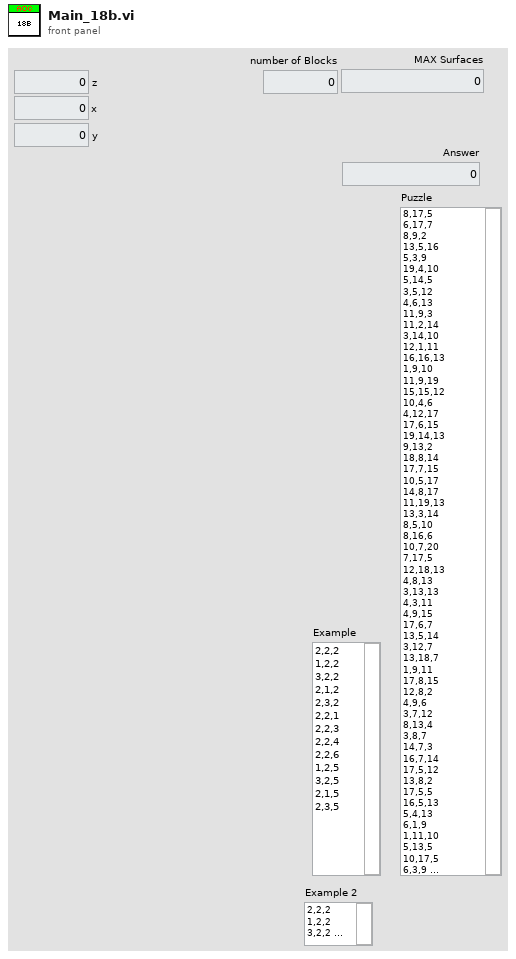
[diagram p1: front panel]
types:
  T1 = typedef "Cluster_Location.ctl" = cluster{"Z":i32, "X":i32, "Y":i32}
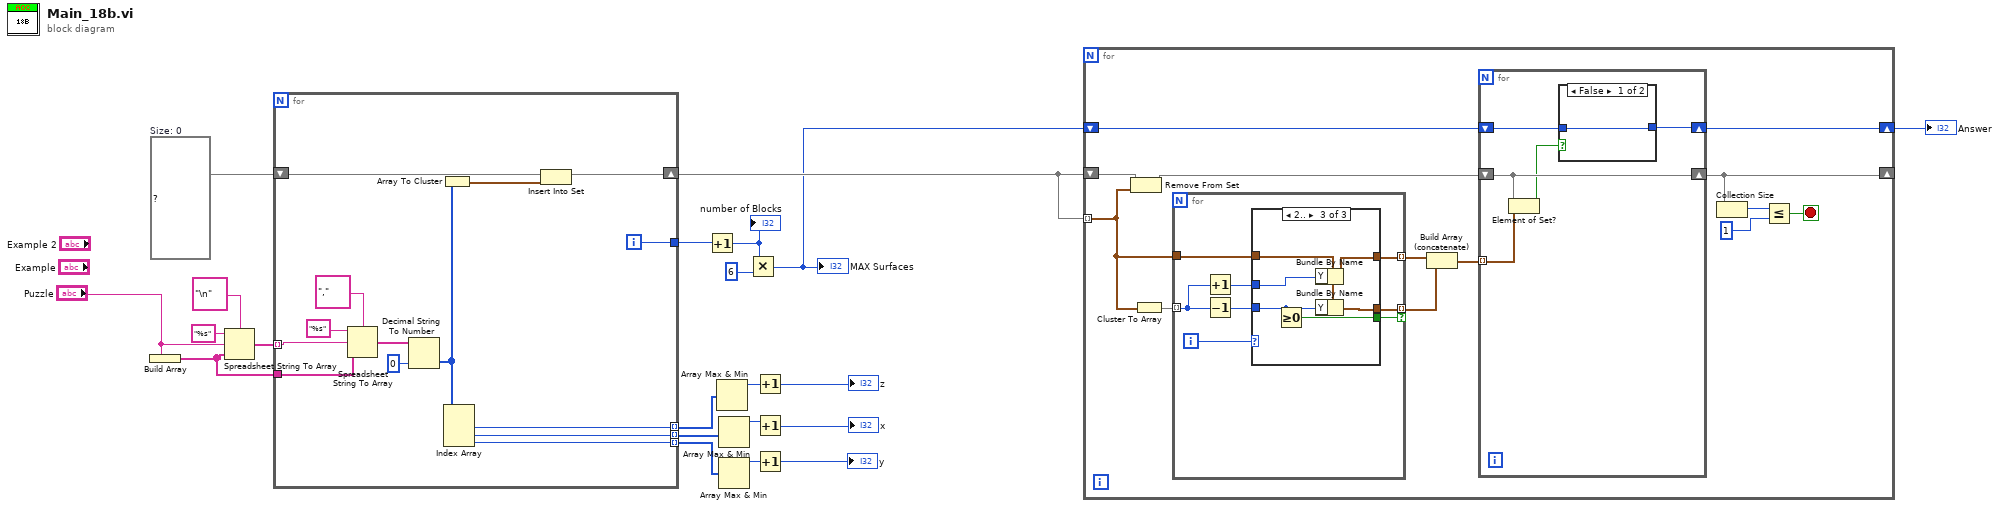
[diagram p0: block diagram]
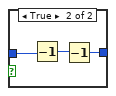
[diagram p2: hidden frame]
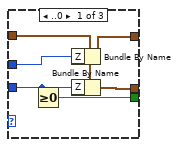
[diagram p3: hidden frame]
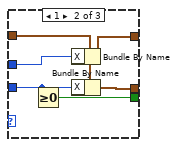
[diagram p4: hidden frame]
diagram:
  w5 = set{T1} {}  # Size: 0
  n1 = Build Array("Puzzle") -> (w18:string[])
  n2 = Spreadsheet String To Array(delimiter (Tab)="\n", format string="%s", spreadsheet string="Puzzle", array type (2D Dbl)=w18) -> (array=w19:string[])
  n3 = for {
    tunnel: w19 -> [w32] mode=indexing
    tunnel: w18 -> [w33]
    tunnel: [w29] -> w17 mode=indexing
    tunnel: [w28] -> w16 mode=indexing
    tunnel: [w27] -> w15 mode=indexing
    tunnel: [w26] -> w7
    shift-right: [w23] -> w4
    shift-left: w5 -> [w24]
    i -> [w26]
    n4 = Spreadsheet String To Array(delimiter (Tab)=",", format string="%s", spreadsheet string=w32, array type (2D Dbl)=w33) -> (array=w30:string[])
    n5 = Decimal String To Number(string=w30, default (0L)=0 ("default (0 I32)")) -> (number=w25:i32[])  [unwired: 1 in, 1 out]
    n6 = Array To Cluster(array=w25) -> (cluster=w22:cluster{"[0]":i32, "[1]":i32, "[2]":i32})
    n7 = Index Array(array=w25) -> (element #1=w29:i32, element #2=w28:i32, element #3=w27:i32)  [unwired: 3 in]
    n8 = Insert Into Set(10:w22, 11:w24) -> (3:w23:set{T1})  [unwired: 1 out]
  }
  n9 = Increment(x=w7) -> (x+1=w6:i32)
  "number of Blocks" <- w6
  n10 = Array Max & Min(array=w17) -> (max value=w14:i32)  [unwired: 3 out]
  n11 = Array Max & Min(array=w16) -> (max value=w13:i32)  [unwired: 3 out]
  n12 = Array Max & Min(array=w15) -> (max value=w12:i32)  [unwired: 3 out]
  n13 = Multiply(x=w6, y=6) -> (x*y=w3:i32)
  "MAX Surfaces" <- w3
  n14 = Increment(x=w14) -> (x+1=→"z":i32)
  n15 = Increment(x=w13) -> (x+1=→"x":i32)
  n16 = Increment(x=w12) -> (x+1=→"y":i32)
  n17 = for {
    shift-right: [w39] -> _
    shift-left: w4 -> [w48]
    tunnel: w4 -> [w46] mode=indexing
    shift-right: [w40] -> w2
    shift-left: w3 -> [w41]
    stop <- w36 stop-if-true
    n18 = Remove From Set(10:w46, 11:w48) -> (3:w42:set{T1})  [unwired: 1 out]
    n19 = Cluster To Array(cluster=w46) -> (array=w47:i32[])
    n20 = for {
      tunnel: w47 -> [w63] mode=indexing
      tunnel: w46 -> [w64]
      tunnel: [w60] -> w45 mode=indexing
      tunnel: [w59] -> w44 mode=indexing if=w58
      i -> [w65]
      n21 = Increment(x=w63) -> (x+1=w61:i32)
      n22 = Decrement(x=w63) -> (x-1=w62:i32)
      n23 = case shown="2.." w65 {
        tunnel: w64 -> [w68 w74 w80]
        tunnel: w62 -> [w69 w75 w81]
        tunnel: w61 -> [w71 w77 w83]
        tunnel: [w70 w76 w82] -> w60
        tunnel: [w67 w73 w79] -> w59
        tunnel: [w66 w72 w78] -> w58
        frame ..0 {
          n24 = Greater Or Equal To 0?(x=w69) -> (x >= 0?=w66:bool)
          n25 = Bundle By Name(cluster=w68, "Z"=w71) -> (w70:T1)
          n26 = Bundle By Name(cluster=w68, "Z"=w69) -> (w67:T1)
        }
        frame 1 {
          n27 = Greater Or Equal To 0?(x=w75) -> (x >= 0?=w72:bool)
          n28 = Bundle By Name(cluster=w74, "X"=w77) -> (w76:T1)
          n29 = Bundle By Name(cluster=w74, "X"=w75) -> (w73:T1)
        }
        frame 2.. {
          n30 = Greater Or Equal To 0?(x=w81) -> (x >= 0?=w78:bool)
          n31 = Bundle By Name(cluster=w80, "Y"=w83) -> (w82:T1)
          n32 = Bundle By Name(cluster=w80, "Y"=w81) -> (w79:T1)
        }
      }
    }
    n33 = Build Array (concatenate)(w45, w44) -> (w43:T1[])
    n34 = for {
      tunnel: w43 -> [w53] mode=indexing
      shift-right: [w52] -> w39
      shift-left: w42 -> [w52]
      shift-right: [w49] -> w40
      shift-left: w41 -> [w50]
      n35 = Element of Set?(10:w53, 11:w52) -> (3:w51:bool)
      n36 = case shown="False" w51 {
        tunnel: w50 -> [w54 w57]
        tunnel: [w54 w55] -> w49
        frame False {
        }
        frame True {
          n37 = Decrement(x=w57) -> (x-1=w56:i32)
          n38 = Decrement(x=w56) -> (x-1=w55:i32)
        }
      }
    }
    n39 = Collection Size(1:w39) -> (0:w38:i32)
    n40 = Less Or Equal?(x=w38, y=1) -> (x <= y?=w36:bool)
  }
  "Answer" <- w2
